vi "RT Microprocessor.vi"() -> ()   [LabVIEW 2014]
doc: "This is the primary Real-Time VI."
uses:
  <vilib>/FPGAPlugInAG/sbRIO-9636/niLvFpga_Open_sbRIO-9636.vi
  <vilib>/rvi/interface/common/dynamic/niFpgaDynamicAddResources.vi
  <vilib>/FPGAPlugInAG/Dynamic/niLvFpga_Reset_Dynamic.vi
  <vilib>/FPGAPlugInAG/Dynamic/niLvFpga_Run_Dynamic.vi
  <vilib>/Utility/error.llb/Error Cluster From Error Code.vi
  <vilib>/rvi/errors/niLvFpgaAdjustHostInterfaceError.vi
  <vilib>/EmbeddedDisplay/Hitachi HD44780/Host/Public/Output (String).vi
  <vilib>/FPGAPlugInAG/Dynamic/niLvFpga_Close_Dynamic.vi
  <vilib>/rvi/interface/nirviOpenFPGA/nirviOpenFPGA.xnode
  FPGA Bitfiles/Exercise5-Window_FPGATarget_Exercise5Solutio_5E92EFA7.lvbitx
  <vilib>/rvi/interface/nirviMethod/nirviMethod.xnode
  <vilib>/rvi/interface/nirviReadWriteControl/nirviReadWriteControl.xnode
  <vilib>/rvi/interface/nirviCloseFPGA/nirviCloseFPGA.xnode
  <vilib>/EmbeddedDisplay/Hitachi HD44780/Host/HD44780 Host.lvlib
  <vilib>/rvi/interface/Simulation/niFpgaSimulationCallBeginRW.vi
  NiFpgaLv.dll
panel:
  out "error out":errorcluster
  in  "Max Temp":fxp<+/-,32,13>=33.0
  out "RPM":fxp<+,32,16>
  out "Temp":fxp<+/-,32,13>
  out "Voltage":fxp<+/-,24,5>
  out "Battery State":enum16{"Charged", "Running", "Low Batt"}(ring)
  out "Temp Warning":bool
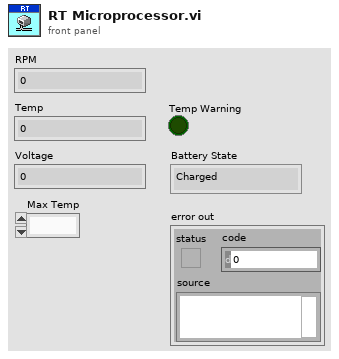
[diagram p1: front panel]
types:
  T1 = enum8{"5x8 & 2 lines", "5x10 & 1 line", "5x8 & 1 line"}
  T2 = enum8{"8x1", "8x2", "12x4", "16x1", "16x2", "16x4", "20x1", "20x2", "20x4", "24x1", "24x2", "40x2", "40x4"}
  T3 = enum16{"Battery State", "RPM", "Temp", "Voltage"}
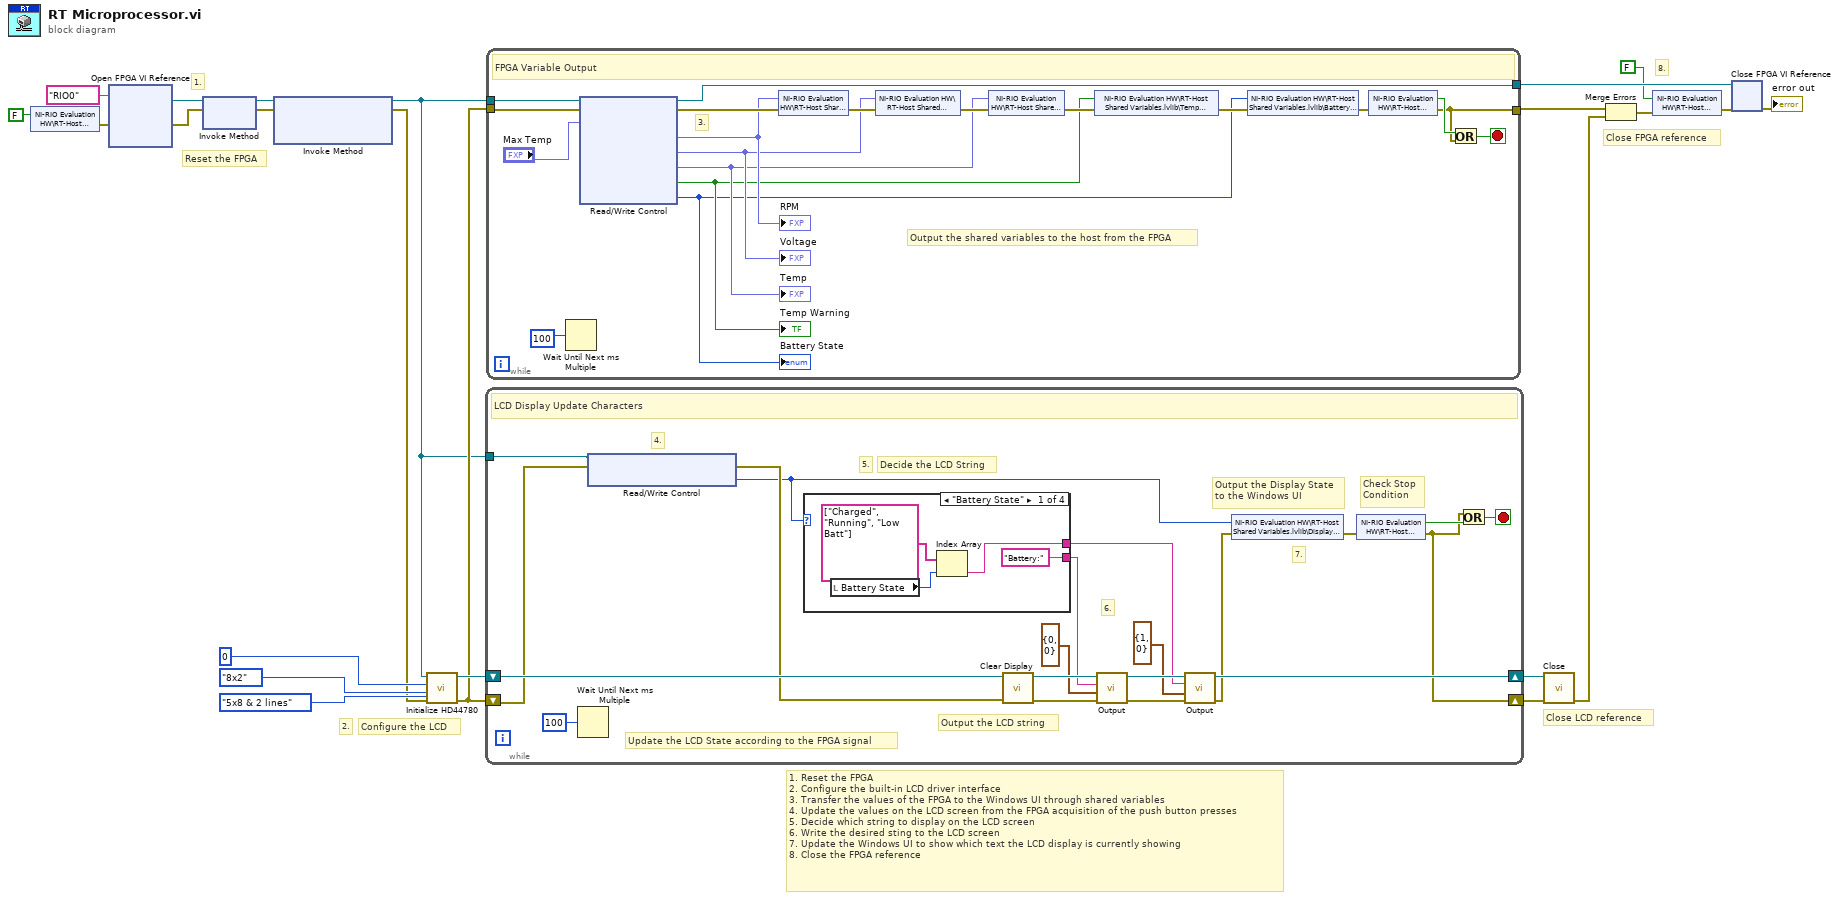
[diagram p0: block diagram]
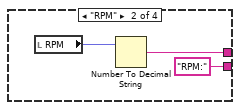
[diagram p2: hidden frame]
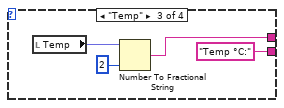
[diagram p3: hidden frame]
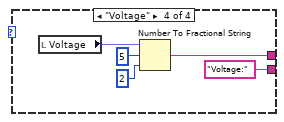
[diagram p4: hidden frame]
diagram:
  # "1. Reset the FPGA\n2. Configure the built-in LCD driver interface\n3. Transfer the values of the FPGA to the Windows UI through shared variables\n4. Update the values on the LCD screen from the FPGA acquisition of the push button presses \n5. Decide which string to display on the LCD screen\n6. Write the desired sting to the LCD screen\n7. Update the Windows UI to show which text the LCD display is currently showing\n8. Close the FPGA reference"
  # "8."
  # "2."
  # "1."
  # "Close FPGA reference"
  # "Close LCD reference"
  # "Configure the LCD"
  # "Reset the FPGA"
  n1 = shared-variable "NI-RIO Evaluation HW\\RT-Host Shared Variables.lvlib\\Stop"(FALSE ("Stop")) -> (error out=w6:errorcluster)  [unwired: 1 in]
  n2 = xnode "Open FPGA VI Reference"("error in"=w6, "resource name"=tag "RIO0") -> ("FPGA VI Reference Out"=w13:refnum<k20>, "error out"=w12:errorcluster)
  n3 = xnode "Invoke Method"("FPGA VI Reference In"=w13, "error in"=w12) -> ("FPGA VI Reference Out"=w11:refnum<k20>, "error out"=w10:errorcluster)
  n4 = xnode "Invoke Method"("FPGA VI Reference In"=w11, "error in"=w10) -> ("FPGA VI Reference Out"=w9:refnum<k20>, "error out"=w8:errorcluster)  [unwired: 1 in]
  n5 = call <vilib>:"Initialize HD44780.vi"("font configuration (5x8 & 2 lines)"=T1."5x8 & 2 lines", "error in (no error)"=w8, "screen size"=T2."8x2", "device index"=i8 0, "FPGA VI Reference in"=w9) -> ("error out"=w18:errorcluster, "LCD out"=w19:refnum<class "Character LCD.lvclass">)  [unwired: 5 in]
  n6 = while {
    shift-right: [w37] -> w17
    shift-left: w19 -> [w38]
    shift-right: [w24] -> w16
    shift-left: w18 -> [w30]
    tunnel: w9 -> [w31]
    stop <- w27 stop-if-true
    # "Check Stop\nCondition"
    # "LCD Display Update Characters"
    # "7."
    # "6."
    # "5."
    # "4."
    # "Output the Display State\nto the Windows UI"
    # "Update the LCD State according to the FPGA signal"
    # "Decide the LCD String"
    # "Output the LCD string"
    n7 = Wait Until Next ms Multiple(millisecond multiple=u32 100) -> ()  [unwired: 1 out]
    n8 = xnode "Read/Write Control"("FPGA VI Reference In"=w31, "error in"=w30) -> ("error out"=w29:errorcluster, "FPGA Display Command"=w28:T3)  [unwired: 1 out]
    n9 = case shown="\"Battery State\"" w28 {
      tunnel: ["Battery:" "RPM:" "Temp °C:" "Voltage:"] -> w39
      tunnel: [w46 w49 w52 w57] -> w32
      frame "Battery State" {
        n10 = local read "Battery State"() -> (w45:enum16{"Charged", "Running", "Low Batt"})
        n11 = Index Array(array=string[] ["Charged", "Running", "Low Batt"], index=w45) -> (element=w46:string)
      }
      frame "RPM" {
        n12 = local read "RPM"() -> (w48:fxp<+,32,16>)
        n13 = Number To Decimal String(number=w48) -> (decimal integer string=w49:string)  [unwired: 1 in]
      }
      frame "Temp" {
        n14 = local read "Temp"() -> (w51:fxp<+/-,32,13>)
        n15 = Number To Fractional String(number=w51, precision (6)=i16 2) -> (F-format string=w52:string)  [unwired: 2 in]
      }
      frame "Voltage" {
        n16 = local read "Voltage"() -> (w55:fxp<+/-,24,5>)
        n17 = Number To Fractional String(number=w55, width (-)=i16 5, precision (6)=i16 2) -> (F-format string=w57:string)  [unwired: 1 in]
      }
    }
    n18 = call <vilib>:"Clear Display.vi"("error in (no error)"=w29, "LCD in"=w38) -> ("error out"=w41:errorcluster, "LCD out"=w40:refnum<class "Character LCD.lvclass">)  [unwired: 8 in]
    n19 = call-poly <vilib>:"Output.vi"("error in (no error)"=w41, "position"=cluster{"row":i8, "column":i8} {"row"=0, "column"=0}, "text"=w39, "LCD in"=w40) -> ("error out"=w43:errorcluster, "LCD out"=w42:refnum<class "Character LCD.lvclass">)  [unwired: 5 in, 1 out]
    n20 = call-poly <vilib>:"Output.vi"("error in (no error)"=w43, "position"=cluster{"row":i8, "column":i8} {"row"=1, "column"=0}, "text"=w32, "LCD in"=w42) -> ("error out"=w33:errorcluster, "LCD out"=w37:refnum<class "Character LCD.lvclass">)  [unwired: 5 in, 1 out]
    n21 = shared-variable "NI-RIO Evaluation HW\\RT-Host Shared Variables.lvlib\\Display State"(w28, error in=w33) -> (error out=w25:errorcluster)
    n22 = shared-variable "NI-RIO Evaluation HW\\RT-Host Shared Variables.lvlib\\Stop"(error in=w25) -> (w26:bool, error out=w24:errorcluster)
    n23 = Or(x=w24, y=w26) -> (x .or. y?=w27:bool)
  }
  n24 = while {
    tunnel: w18 -> [w78]
    tunnel: [w77] -> w23
    tunnel: [w60] -> w15
    tunnel: w9 -> [w64]
    stop <- w63 stop-if-true
    # "FPGA Variable Output"
    # "3."
    # "Output the shared variables to the host from the FPGA"
    n25 = Wait Until Next ms Multiple(millisecond multiple=u32 100) -> ()  [unwired: 1 out]
    n26 = xnode "Read/Write Control"("FPGA VI Reference In"=w64, "error in"=w78, "Max Temp"="Max Temp") -> ("FPGA VI Reference Out"=w77:refnum<k20>, "error out"=w72:errorcluster, "RPM"=w69:fxp<+,32,16>, "Voltage"=w68:fxp<+/-,24,5>, "Temp"=w67:fxp<+/-,32,13>, "Temp Warning"=w66:bool, "Battery State"=w65:enum16{"Charged", "Running", "Low Batt"})
    "Temp Warning" <- w66
    "Battery State" <- w65
    "Voltage" <- w68
    "Temp" <- w67
    "RPM" <- w69
    n27 = shared-variable "NI-RIO Evaluation HW\\RT-Host Shared Variables.lvlib\\RPM"(w69, error in=w72) -> (error out=w73:errorcluster)
    n28 = shared-variable "NI-RIO Evaluation HW\\RT-Host Shared Variables.lvlib\\Voltage"(w68, error in=w73) -> (error out=w75:errorcluster)
    n29 = shared-variable "NI-RIO Evaluation HW\\RT-Host Shared Variables.lvlib\\Temp"(w67, error in=w75) -> (error out=w71:errorcluster)
    n30 = shared-variable "NI-RIO Evaluation HW\\RT-Host Shared Variables.lvlib\\Temp Warning"(w66, error in=w71) -> (error out=w70:errorcluster)
    n31 = shared-variable "NI-RIO Evaluation HW\\RT-Host Shared Variables.lvlib\\Battery State"(w65, error in=w70) -> (error out=w62:errorcluster)
    n32 = shared-variable "NI-RIO Evaluation HW\\RT-Host Shared Variables.lvlib\\Stop"(error in=w62) -> (w61:bool, error out=w60:errorcluster)
    n33 = Or(x=w61, y=w60) -> (x .or. y?=w63:bool)
  }
  n34 = call <vilib>:"Close.vi"("error in (no error)"=w16, "LCD in"=w17) -> ("error out"=w7:errorcluster)  [unwired: 9 in]
  n35 = Merge Errors(w15, w7) -> (w3:errorcluster)
  n36 = shared-variable "NI-RIO Evaluation HW\\RT-Host Shared Variables.lvlib\\Stop"(FALSE ("Stop"), error in=w3) -> (error out=w2:errorcluster)
  n37 = xnode "Close FPGA VI Reference"("FPGA VI Reference In"=w23, "error in"=w2) -> ("error out"=→"error out":errorcluster)
